vi "DSF.Memory.Cache.Transfer.Get Channel Configuration.vi"(8 "error in (no error)":errorcluster, 11 "Transfer Cache in":refnum<class "DSF.Memory.Cache.Transfer.lvclass">) -> (0 "error out":errorcluster, 2 "Channel Configuration":T1[](array[typedef]) {"count" format="%d elements"; "offset" format="%d bytes"}, 3 "Transfer Cache out":refnum<class "DSF.Memory.Cache.Transfer.lvclass">)   [LabVIEW 2016, in "DSF.Memory.lvlib" / "DSF.Memory.Cache.Transfer.lvclass"]
uses:
  DSF.Memory.Cache.Transfer.lvclass
  Typedefs/DSF.Memory.Buffer Channel Configuration.ctl
  Typedefs/DSF.Common.Data Type.ctl
  DSF.Memory.Cache.Transfer.lvclass/DSF.Memory.Cache.Transfer.ctl
  DSF.Common.lvlib
  DSF.Memory.lvlib
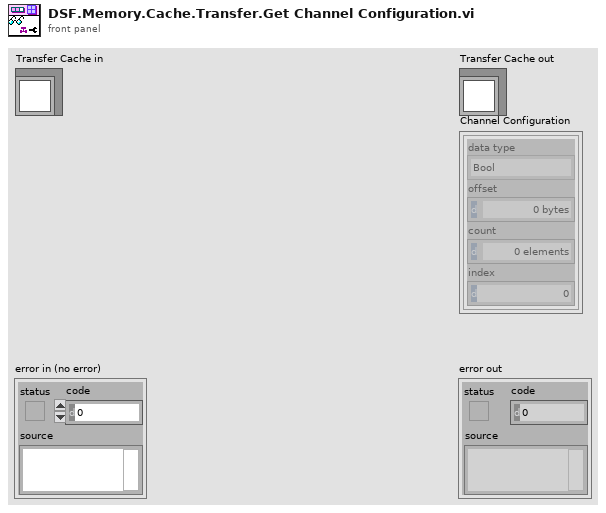
[diagram p1: front panel]
types:
  T1 = typedef "DSF.Memory.lvlib/DSF.Memory.Buffer Channel Configuration.ctl" = cluster{"data type":T2, "offset":u64, "count":u64, "index":u64}
  T2 = typedef "DSF.Common.lvlib/DSF.Common.Data Type.ctl" = enum8{"Bool", "SGL", "DBL", "I8", "I16", "I32", "I64", "U8", "U16", "U32", "U64"}
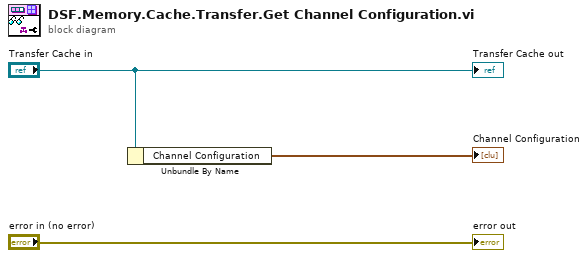
[diagram p0: block diagram]
diagram:
  n1 = Unbundle By Name("Transfer Cache in") -> ("Channel Configuration"=→"Channel Configuration":T1[])
  "error out" <- "error in (no error)"
  "Transfer Cache out" <- "Transfer Cache in"
